vi "Get stack cell d_voltage status.vi"(10 "Dilico Measurement Controls":T1={"Number of cells"=10, "Wait time [ms]"=20.0, "UnderVoltage Limit [mV]"=700, "OverVoltage Limit [mV]"=2000} {"OverVoltage Limit [mV]" max=5000 step=1; "Wait time [ms]" min=0 max=25.5; "UnderVoltage Limit [mV]" max=5000 step=1}, 11 "Status Map":map{string, dbl}(c390)) -> (0 "CVM":cluster{i32[], dbl[]}[](graph), 1 "Min":dbl, 2 "Max":dbl, 3 "Sum Stack V":dbl, 4 "Average":dbl, 5 "Cell(s) OV":string, 6 "Plot(s)":i32, 7 "Cell(s) UV":string)   [LabVIEW 2025, in "phlair-busch-can-bus.lvlib"]
uses:
  DilicoControls.ctl
  <vilib>/Utility/error.llb/Trim Whitespace One-Sided.vi
  <userlib>/_MGI/1D Array/MGI Average/MGI Average (DBL[]).vi
  phlair-busch-can-bus.lvlib
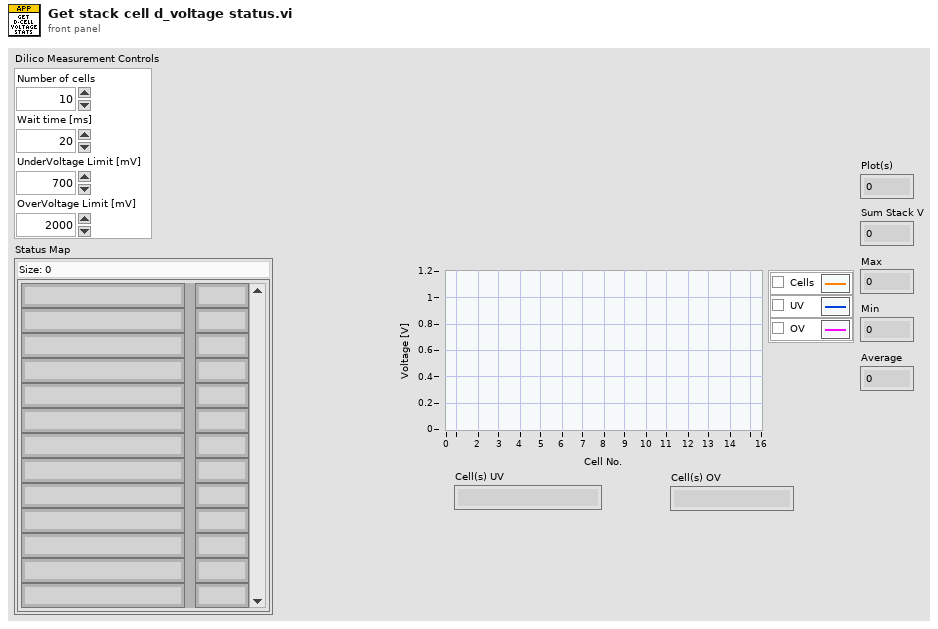
[diagram p1: front panel]
types:
  T1 = typedef "phlair-busch-can-bus.lvlib/DilicoControls.ctl" = cluster{"Number of cells":u8, "Wait time [ms]":sgl, "UnderVoltage Limit [mV]":u16, "OverVoltage Limit [mV]":u16}
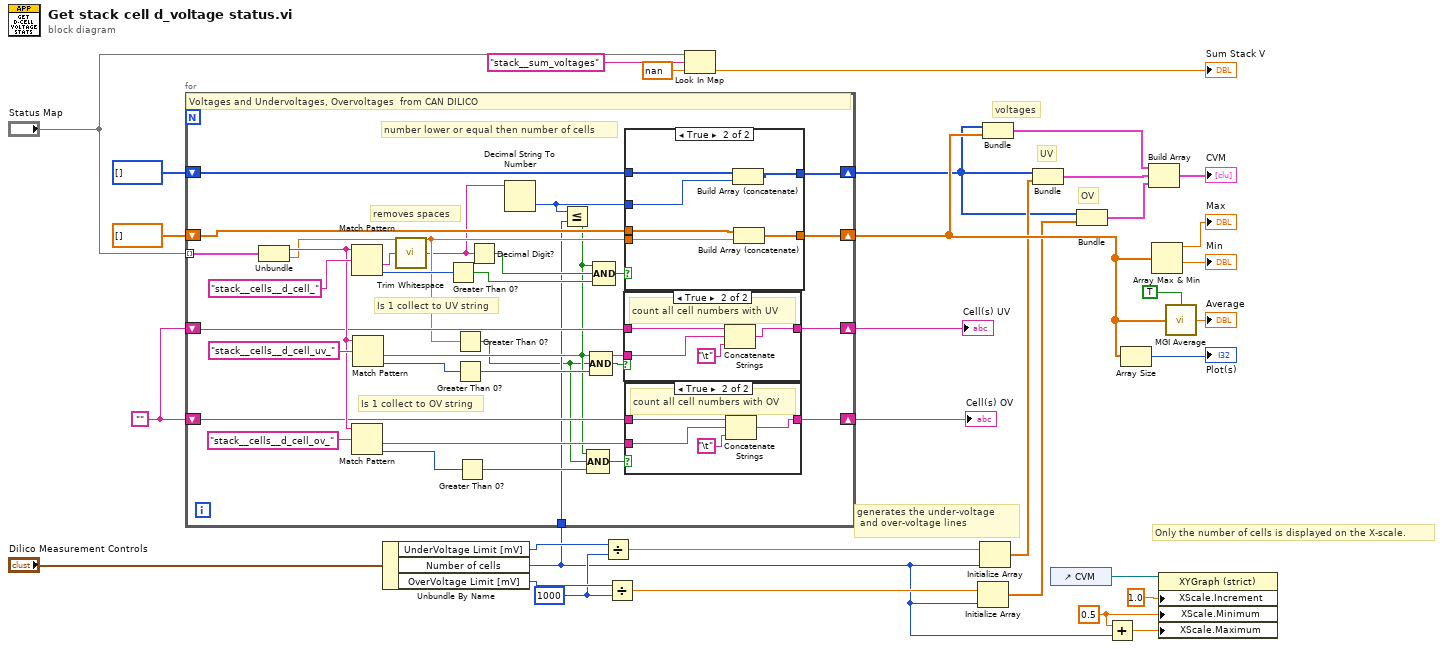
[diagram p0: block diagram]
diagram:
  w6 = u16 1000 ("y")
  w18 = ""
  w3 = 0.5 ("X Scale.Range:Minimum")
  # "Only the number of cells is displayed on the X-scale."
  # "OV"
  # "UV"
  # "voltages"
  # "generates the under-voltage\n and over-voltage lines"
  n1 = Unbundle By Name("Dilico Measurement Controls") -> ("UnderVoltage Limit [mV]"=w5:u16, "Number of cells"=w1:u8, "OverVoltage Limit [mV]"=w8:u16)
  n2 = for {
    tunnel: "Status Map" -> [w65] mode=indexing
    shift-right: [w61] -> w11
    shift-left: i32[] [] -> [w58]
    shift-right: [w60] -> w20
    shift-left: dbl[] [] -> [w59]
    shift-right: [w53] -> w16
    shift-left: w18 -> [w52]
    shift-right: [w50] -> w17
    shift-left: w18 -> [w49]
    tunnel: w1 -> [w37]
    # "number lower or equal then number of cells"
    # "Is 1 collect to OV string"
    # "Is 1 collect to UV string"
    # "removes spaces"
    # "Voltages and Undervoltages, Overvoltages  from CAN DILICO"
    n3 = Unbundle(w65) -> (w55:string, w42:dbl)
    n4 = Match Pattern(string=w55, regular expression="stack__cells__d_cell_") -> (after substring=w40:string, offset past match=w62:i32)  [unwired: 1 in, 2 out]
    n5 = Match Pattern(string=w55, regular expression="stack__cells__d_cell_ov_") -> (after substring=w54:string, offset past match=w41:i32)  [unwired: 1 in, 2 out]
    n6 = Match Pattern(string=w55, regular expression="stack__cells__d_cell_uv_") -> (after substring=w51:string, offset past match=w35:i32)  [unwired: 1 in, 2 out]
    n7 = call <vilib>:"Trim Whitespace.vi"("string"=w40) -> ("trimmed string"=w39:string)  [unwired: 1 in]
    n8 = Greater Than 0?(x=w62) -> (x > 0?=w64:bool)
    n9 = Greater Than 0?(x=w42) -> (x > 0?=w34:bool)
    n10 = Greater Than 0?(x=w35) -> (x > 0?=w45:bool)
    n11 = Greater Than 0?(x=w41) -> (x > 0?=w44:bool)
    n12 = Decimal Digit?(1:w39) -> (0:w47:bool)
    n13 = Decimal String To Number(string=w39) -> (number=w38:i32)  [unwired: 2 in, 1 out]
    n14 = Less Or Equal?(x=w38, y=w37) -> (x <= y?=w36:bool)
    n15 = Compound Arithmetic op=AND(w36, w34, w44) -> (w43:bool)
    n16 = Compound Arithmetic op=AND(w36, w34, w45) -> (w46:bool)
    n17 = Compound Arithmetic op=AND(w36, w47, w64) -> (w48:bool)
    n18 = case shown="True" w46 {
      tunnel: w51 -> [_ w69]
      tunnel: [w66 w70] -> w50
      tunnel: w49 -> [w66 w68]
      frame False {
      }
      frame True {
        # "count all cell numbers with UV"
        n19 = Concatenate Strings(w68, w69, "\t") -> (w70:string)
      }
    }
    n20 = case shown="True" w48 {
      tunnel: w42 -> [_ w83]
      tunnel: [w77 w82] -> w61
      tunnel: [w76 w81] -> w60
      tunnel: w59 -> [w76 w80]
      tunnel: w58 -> [w77 w79]
      tunnel: w38 -> [_ w78]
      frame False {
      }
      frame True {
        n21 = Build Array (concatenate)(w79, w78) -> (w82:i32[])
        n22 = Build Array (concatenate)(w80, w83) -> (w81:dbl[])
      }
    }
    n23 = case shown="True" w43 {
      tunnel: w54 -> [_ w74]
      tunnel: [w71 w75] -> w53
      tunnel: w52 -> [w71 w73]
      frame False {
      }
      frame True {
        # "count all cell numbers with OV"
        n24 = Concatenate Strings(w73, w74, "\t") -> (w75:string)
      }
    }
  }
  "Cell(s) UV" <- w17
  "Cell(s) OV" <- w16
  n25 = Divide(x=w5, y=w6) -> (x/y=w4:dbl)
  n26 = Divide(x=w8, y=w6) -> (x/y=w7:dbl)
  n27 = Look In Map(map="Status Map", key="stack__sum_voltages", default value=nan) -> (value=→"Sum Stack V":dbl)  [unwired: 1 out]
  n28 = Initialize Array(w7, w1) -> (w10:dbl[])
  n29 = Initialize Array(w4, w1) -> (w13:dbl[])
  n30 = Bundle(w11, w20) -> (w19:cluster{i32[], dbl[]})  [unwired: 1 in]
  n31 = Bundle(w11, w13) -> (w14:cluster{i32[], dbl[]})  [unwired: 1 in]
  n32 = control-ref of="CVM"() -> (w26:refnum<vi>)
  n33 = Bundle(w11, w10) -> (w12:cluster{i32[], dbl[]})  [unwired: 1 in]
  n34 = Add(x=w3, y=w1) -> (x+y=w2:dbl)
  n35 = Array Size(array=w20) -> (size(s)=→"Plot(s)":i32)
  n36 = Build Array(w19, w14, w12) -> (→"CVM":cluster{i32[], dbl[]}[])
  n37 = Array Max & Min(array=w20) -> (max value=→"Max":dbl, min value=→"Min":dbl)  [unwired: 2 out]
  n38 = property class="XYGraph (strict)"(reference=w26, "XScale.Increment"=1.0 ("X Scale.Range:Increment"), "XScale.Minimum"=w3, "XScale.Maximum"=w2) -> ()  [unwired: 1 in, 2 out]
  n39 = call-poly <userlib>:"MGI Average.vi"("Double[]"=w20, "Ignore NaN? (F)"=TRUE) -> ("Average"=→"Average":dbl)
